vi "Create Plane Object.vi"(7 "Plane":enum16{"X-Y Plane", "Y-Z Plane", "X-Z Plane"}(ring), 8 "error in (no error)":errorcluster, 9 "Offset":sgl, 10 "RGBA":cluster{"R":sgl, "G":sgl, "B":sgl, "A":sgl}, 11 "Range Cluster":T1) -> (0 "error out":errorcluster, 3 "Cursor Plane Object":refnum<vi>)   [LabVIEW 2017, in "3D Plot.lvclass"]
uses:
  <vilib>/Math Plots/3D Math Plots/3D Plot/3D Plot/3D Plot.lvclass
  <vilib>/picture/3D Picture Control/Object/Create Object (name).vi
  <vilib>/picture/3D Picture Control/NI_3D Picture Control.lvlib
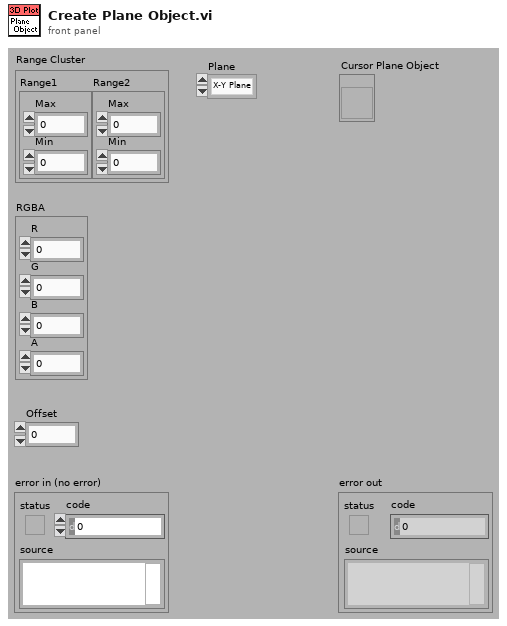
[diagram p1: front panel]
types:
  T1 = cluster{"Range1":cluster{"Max":sgl, "Min":sgl}, "Range2":cluster{"Max":sgl, "Min":sgl}}
  T2 = enum16{"Normal Bin", "Opaque Bin", "Transparent Bin"}
  T3 = enum16{"Overall", "Per Primitive", "Per Vertex", "Binding Off"}
  T4 = enum16{"Points", "Lines", "Line Strip", "Line Loop", "Triangles", "Triangle Strip", "Triangle Fan", "Quads", "Quad Strip", "Polygon"}
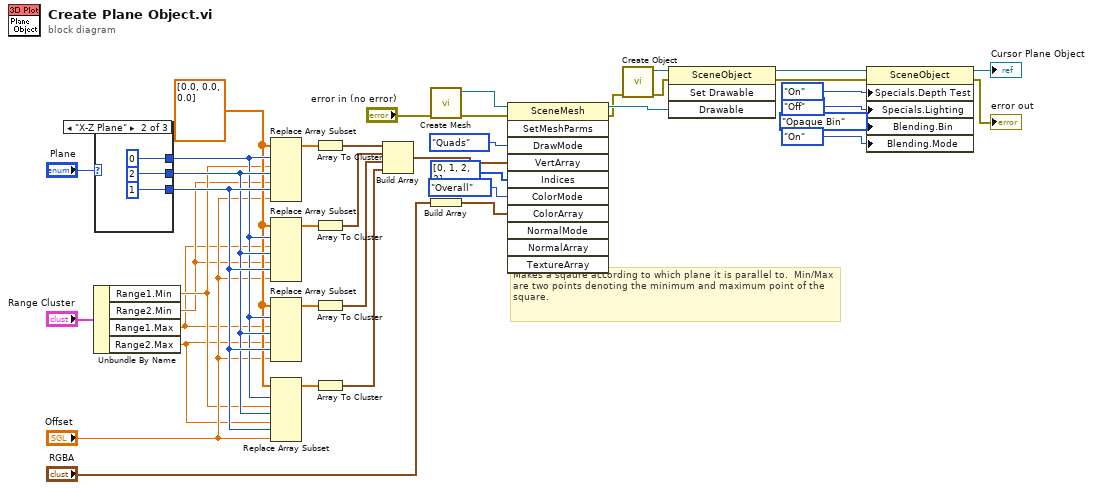
[diagram p0: block diagram]
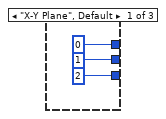
[diagram p2: hidden frame]
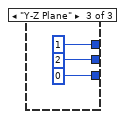
[diagram p3: hidden frame]
diagram:
  w29 = sgl[] [0.0, 0.0, 0.0]
  # "Makes a sqaure according to which plane it is parallel to.  Min/Max are two points denoting the minimum and maximum point of the square."
  n1 = Unbundle By Name("Range Cluster") -> ("Range1.Min"=w26:sgl, "Range2.Min"=w25:sgl, "Range1.Max"=w24:sgl, "Range2.Max"=w23:sgl)
  n2 = case shown="\"X-Z Plane\"" "Plane" {
    tunnel: [0 0 1] -> w30
    tunnel: [1 2 2] -> w31
    tunnel: [2 1 0] -> w32
    frame "X-Y Plane", Default {
    }
    frame "X-Z Plane" {
    }
    frame "Y-Z Plane" {
    }
  }
  n3 = Replace Array Subset(array=w29, new element #1=w26, index #1=w30, new element #2=w25, index #2=w31, new element #3="Offset", index #3=w32) -> (w33:sgl[])
  n4 = Replace Array Subset(array=w29, new element #1=w24, index #1=w30, new element #2=w25, index #2=w31, new element #3="Offset", index #3=w32) -> (w34:sgl[])
  n5 = Replace Array Subset(array=w29, new element #1=w24, index #1=w30, new element #2=w23, index #2=w31, new element #3="Offset", index #3=w32) -> (w35:sgl[])
  n6 = Replace Array Subset(array=w29, new element #1=w26, index #1=w30, new element #2=w23, index #2=w31, new element #3="Offset", index #3=w32) -> (w36:sgl[])
  n7 = Array To Cluster(array=w33) -> (cluster=w37:cluster{"[0]":sgl, "[1]":sgl, "[2]":sgl})
  n8 = Array To Cluster(array=w34) -> (cluster=w38:cluster{"[0]":sgl, "[1]":sgl, "[2]":sgl})
  n9 = Array To Cluster(array=w35) -> (cluster=w39:cluster{"[0]":sgl, "[1]":sgl, "[2]":sgl})
  n10 = Array To Cluster(array=w36) -> (cluster=w40:cluster{"[0]":sgl, "[1]":sgl, "[2]":sgl})
  n11 = Build Array(w37, w38, w39, w40) -> (w7:cluster{"[0]":sgl, "[1]":sgl, "[2]":sgl}[])
  n12 = call <vilib>:"Create Mesh.vi"("error in (no error)"="error in (no error)") -> ("error out"=w20:errorcluster, "New Mesh Refnum"=w21:refnum<vi>)  [unwired: 9 out]
  n13 = Build Array("RGBA") -> (w6:cluster{"R":sgl, "G":sgl, "B":sgl, "A":sgl}[])
  n14 = invoke class="SceneMesh" method="SetMeshParms"(reference=w21, error in=w20, "DrawMode"=T4."Quads" ("Draw Mode"), "VertArray"=w7, "Indices"=u32[] [0, 1, 2, 3], "ColorMode"=T3."Overall" ("Color Binding Mode"), "ColorArray"=w6) -> (reference out=w16:refnum<vi>, error out=w10:errorcluster)  [unwired: 4 in, 9 out]
  n15 = call-poly <vilib>:"Create Object.vi"("error in (no error)"=w10) -> ("error out"=w9:errorcluster, "Scene:New Object"=w17:refnum<vi>)  [unwired: 9 in]
  n16 = invoke class="SceneObject" method="Set Drawable"(reference=w17, error in=w9, "Drawable"=w16) -> (reference out=w15:refnum<vi>, error out=w8:errorcluster)  [unwired: 1 in, 2 out]
  n17 = property class="SceneObject"(reference=w15, error in=w8, "Specials.Depth Test"=enum16{"Inherit Value", "Off", "On"}."On" ("Specials:Depth Test"), "Specials.Lighting"=enum16{"Inherit Value", "Off", "On"}."Off" ("Specials:Lighting"), "Blending.Bin"=T2."Opaque Bin" ("Blending:Bin"), "Blending.Mode"=enum16{"Inherit Value", "Off", "On"}."On" ("Blending:Mode")) -> (reference out=→"Cursor Plane Object":refnum<vi>, error out=→"error out":errorcluster)
